vi "Apply_f.vi"(4 "w_bar_r":dbl, 6 "w_bar_ca":dbl, 7 "Input State Var":T2, 8 "Alpha_r":dbl, 9 "Alpha_c":dbl, 10 "T":dbl, 11 "Input State":T1) -> (0 "Trend":dbl, 3 "Output State":T1)   [LabVIEW 2019]
uses:
  <vilib>/Analysis/NI_AALBase.lvlib
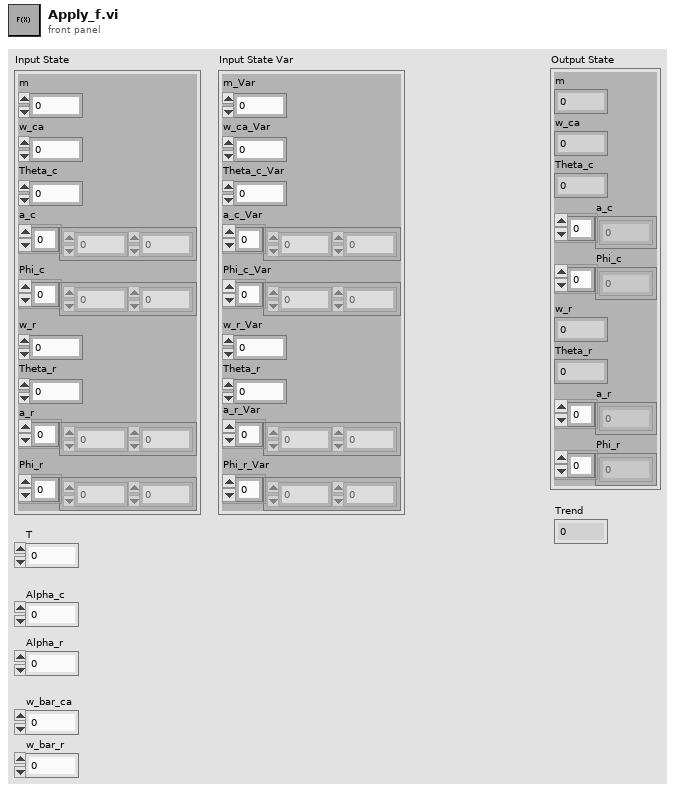
[diagram p1: front panel]
types:
  T1 = cluster{"m":dbl, "w_ca":dbl, "Theta_c":dbl, "a_c":dbl[], "Phi_c":dbl[], "w_r":dbl, "Theta_r":dbl, "a_r":dbl[], "Phi_r":dbl[]}
  T2 = cluster{"m_Var":dbl, "w_ca_Var":dbl, "Theta_c_Var":dbl, "a_c_Var":dbl[], "Phi_c_Var":dbl[], "w_r_Var":dbl, "Theta_r":dbl, "a_r_Var":dbl[], "Phi_r_Var":dbl[]}
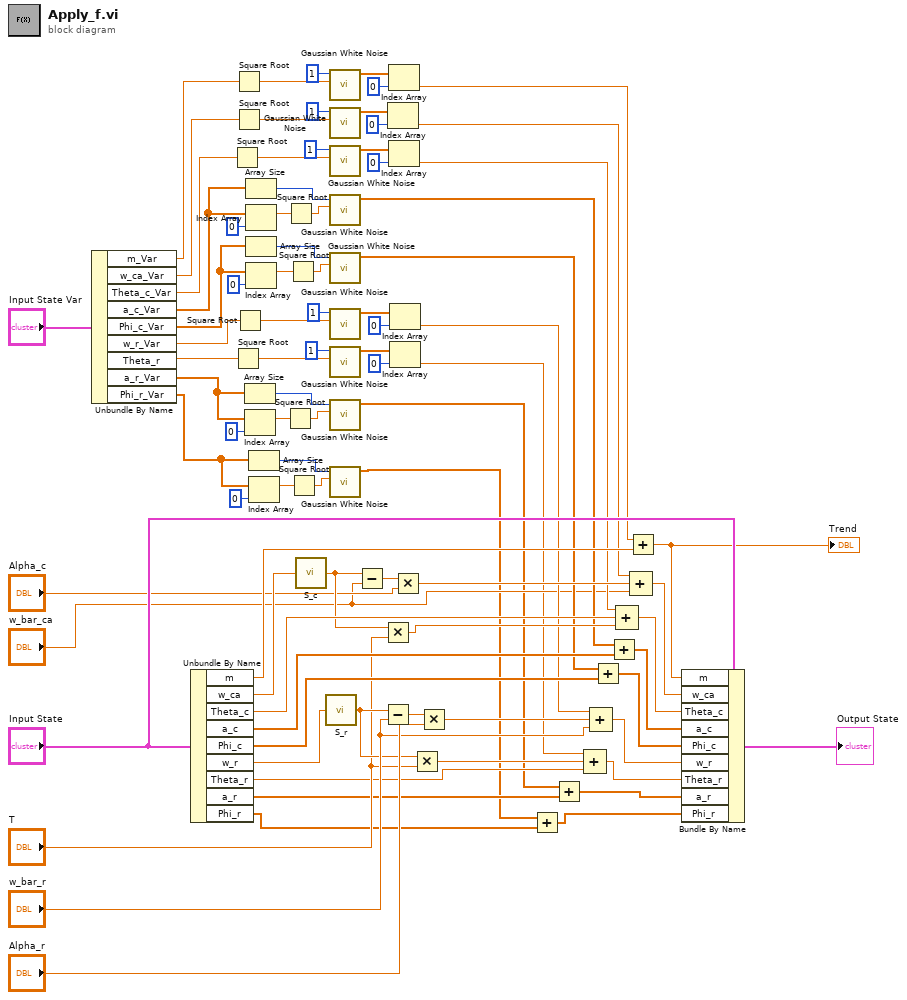
[diagram p0: block diagram]
diagram:
  n1 = Unbundle By Name("Input State Var") -> ("m_Var"=w86:dbl, "w_ca_Var"=w81:dbl, "Theta_c_Var"=w79:dbl, "a_c_Var"=w75:dbl[], "Phi_c_Var"=w68:dbl[], "w_r_Var"=w65:dbl, "Theta_r"=w62:dbl, "a_r_Var"=w57:dbl[], "Phi_r_Var"=w52:dbl[])
  n2 = Unbundle By Name("Input State") -> ("m"=w51:dbl, "w_ca"=w46:dbl, "Theta_c"=w36:dbl, "a_c"=w33:dbl[], "Phi_c"=w27:dbl[], "w_r"=w26:dbl, "Theta_r"=w10:dbl, "a_r"=w6:dbl[], "Phi_r"=w3:dbl[])
  n3 = Square Root(x=w79) -> (sqrt(x)=w80:dbl)
  n4 = Square Root(x=w62) -> (sqrt(x)=w63:dbl)
  n5 = Square Root(x=w86) -> (sqrt(x)=w85:dbl)
  n6 = Square Root(x=w81) -> (sqrt(x)=w82:dbl)
  n7 = Square Root(x=w65) -> (sqrt(x)=w67:dbl)
  n8 = Array Size(array=w57) -> (size(s)=w59:i32)
  n9 = Index Array(array=w57, index=0) -> (element=w60:dbl)
  n10 = Array Size(array=w75) -> (size(s)=w76:i32)
  n11 = Index Array(array=w75, index=0) -> (element=w74:dbl)
  n12 = Array Size(array=w68) -> (size(s)=w70:i32)
  n13 = Index Array(array=w68, index=0) -> (element=w71:dbl)
  n14 = Array Size(array=w52) -> (size(s)=w55:i32)
  n15 = Index Array(array=w52, index=0) -> (element=w54:dbl)
  n16 = Square Root(x=w60) -> (sqrt(x)=w58:dbl)
  n17 = Square Root(x=w74) -> (sqrt(x)=w77:dbl)
  n18 = Square Root(x=w71) -> (sqrt(x)=w69:dbl)
  n19 = Square Root(x=w54) -> (sqrt(x)=w56:dbl)
  n20 = call "S_c.vi"("w_in"=w46) -> ("w_out"=w35:dbl)
  n21 = call "S_r.vi"("w_in"=w26) -> ("w_out"=w16:dbl)
  n22 = call <vilib>:"Gaussian White Noise.vi"("standard deviation"=w85, "samples"=1) -> ("Gaussian noise pattern"=w50:dbl[])  [unwired: 8 in, 1 out]
  n23 = call <vilib>:"Gaussian White Noise.vi"("standard deviation"=w82, "samples"=1) -> ("Gaussian noise pattern"=w42:dbl[])  [unwired: 8 in, 1 out]
  n24 = call <vilib>:"Gaussian White Noise.vi"("standard deviation"=w80, "samples"=1) -> ("Gaussian noise pattern"=w38:dbl[])  [unwired: 8 in, 1 out]
  n25 = call <vilib>:"Gaussian White Noise.vi"("standard deviation"=w77, "samples"=w76) -> ("Gaussian noise pattern"=w32:dbl[])  [unwired: 8 in, 1 out]
  n26 = call <vilib>:"Gaussian White Noise.vi"("standard deviation"=w69, "samples"=w70) -> ("Gaussian noise pattern"=w28:dbl[])  [unwired: 8 in, 1 out]
  n27 = call <vilib>:"Gaussian White Noise.vi"("standard deviation"=w67, "samples"=1) -> ("Gaussian noise pattern"=w21:dbl[])  [unwired: 8 in, 1 out]
  n28 = call <vilib>:"Gaussian White Noise.vi"("standard deviation"=w63, "samples"=1) -> ("Gaussian noise pattern"=w12:dbl[])  [unwired: 8 in, 1 out]
  n29 = call <vilib>:"Gaussian White Noise.vi"("standard deviation"=w58, "samples"=w59) -> ("Gaussian noise pattern"=w7:dbl[])  [unwired: 8 in, 1 out]
  n30 = call <vilib>:"Gaussian White Noise.vi"("standard deviation"=w56, "samples"=w55) -> ("Gaussian noise pattern"=w4:dbl[])  [unwired: 8 in, 1 out]
  n31 = Subtract(x=w35, y="w_bar_ca") -> (x-y=w45:dbl)
  n32 = Multiply(x=w35, y="T") -> (x*y=w34:dbl)
  n33 = Subtract(x=w16, y="w_bar_r") -> (x-y=w25:dbl)
  n34 = Index Array(array=w42, index=0) -> (element=w41:dbl)
  n35 = Index Array(array=w50, index=0) -> (element=w49:dbl)
  n36 = Index Array(array=w38, index=0) -> (element=w37:dbl)
  n37 = Index Array(array=w21, index=0) -> (element=w20:dbl)
  n38 = Index Array(array=w12, index=0) -> (element=w11:dbl)
  n39 = Multiply(x=w45, y="Alpha_c") -> (x*y=w44:dbl)
  n40 = Multiply(x=w16, y="T") -> (x*y=w14:dbl)
  n41 = Multiply(x=w25, y="Alpha_r") -> (x*y=w19:dbl)
  n42 = Add(x=w4, y=w3) -> (x+y=w5:dbl[])
  n43 = Add(x=w7, y=w6) -> (x+y=w8:dbl[])
  n44 = Compound Arithmetic op=ADD(w11, w14, w10) -> (w9:dbl)
  n45 = Compound Arithmetic op=ADD(w20, w19, "w_bar_r") -> (w23:dbl)
  n46 = Add(x=w28, y=w27) -> (x+y=w29:dbl[])
  n47 = Add(x=w32, y=w33) -> (x+y=w31:dbl[])
  n48 = Compound Arithmetic op=ADD(w37, w36, w34) -> (w40:dbl)
  n49 = Add(x=w49, y=w51) -> (x+y=w1:dbl)
  "Trend" <- w1
  n50 = Compound Arithmetic op=ADD(w41, w44, "w_bar_ca") -> (w47:dbl)
  n51 = Bundle By Name(cluster="Input State", "m"=w1, "w_ca"=w47, "Theta_c"=w40, "a_c"=w31, "Phi_c"=w29, "w_r"=w23, "Theta_r"=w9, "a_r"=w8, "Phi_r"=w5) -> (→"Output State":T1)
